vi "Indent String.vi"(1 "Level":i32=1, 3 "String":string="This is a string\nwith multiple lines\nwhich should be indented") -> (0 "Result":string)   [LabVIEW 2018, in "CubeLogger.lvclass"]
uses:
  CubeLogger/CubeLogger.lvclass
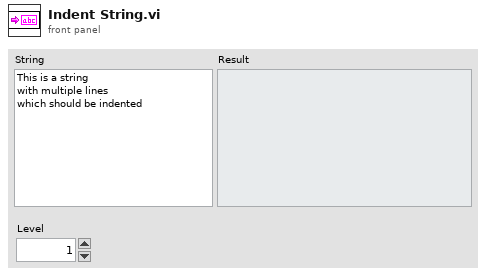
[diagram p1: front panel]
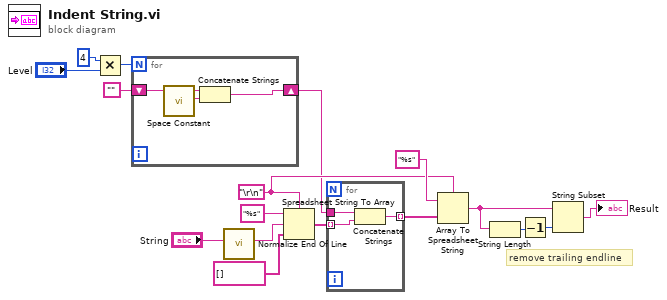
[diagram p0: block diagram]
diagram:
  w10 = "\r\n"
  # "remove trailing endline"
  n1 = Multiply(x=4, y="Level") -> (x*y=w8:i32)
  n2 = for {
    N: w8 -> [_]
    shift-right: [w19] -> w5
    shift-left: "" -> [w20]
    n3 = call <vilib>:"Space Constant.vi"() -> ("String"=w18:string)
    n4 = Concatenate Strings(w20, w18) -> (w19:string)
  }
  n5 = call <vilib>:"Normalize End Of Line.vi"("string in"="String") -> ("string out"=w13:string)  [unwired: 7 in]
  n6 = Spreadsheet String To Array(delimiter (Tab)=w10, format string="%s", spreadsheet string=w13, array type (2D Dbl)=string[] []) -> (array=w15:string[])
  n7 = for {
    tunnel: w15 -> [w23] mode=indexing
    tunnel: [w22] -> w12 mode=indexing
    tunnel: w5 -> [w21]
    n8 = Concatenate Strings(w21, w23) -> (w22:string)
  }
  n9 = Array To Spreadsheet String(delimiter (Tab)=w10, array=w12, 3:"%s" ("format string")) -> (spreadsheet string=w3:string)
  n10 = String Length(string=w3) -> (length=w2:i32)
  n11 = Decrement(x=w2) -> (x-1=w1:i32)
  n12 = String Subset(string=w3, length (rest)=w1) -> (substring=→"Result":string)  [unwired: 1 in]
